vi "Enable pneumatics.vi"(8 "error in":errorcluster, 11 "UTP IO Session in":T1) -> (0 "error out":errorcluster, 3 "UTP IO Session out":T1)   [LabVIEW 2023, in "Actuators.lvlib"]
doc: "Send 1s pulse length to enable all pneumatics"
uses:
  Actuators.lvlib
  <vilib>/Noffz/UTP IO/UTP IO Library/Typedefs/Session Handle.ctl
  <vilib>/Noffz/UTP IO/UTP IO Library/UTP IO Pool Session.lvclass
  c9def3e0-2d72-4d59-8dd4-2fe76db72e2b.vi
  <vilib>/Noffz/UTP IO/UTP IO Library/methods/poly/plc/Write PLC Variable (Boolean).vi
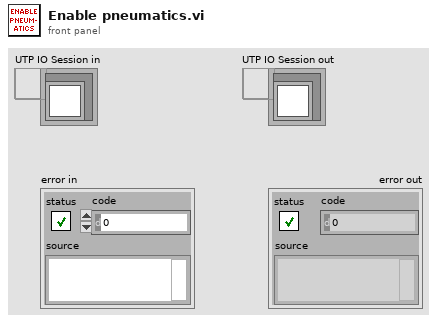
[diagram p1: front panel]
types:
  T1 = typedef "UTP IO Library.lvlib/UTP IO Pool Session.lvclass/Session Handle.ctl" = refnum<data-value>
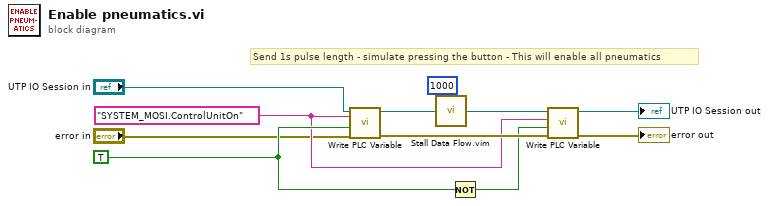
[diagram p0: block diagram]
diagram:
  w4 = TRUE ("value")
  w3 = "SYSTEM_MOSI.ControlUnitOn" ("variable name")
  # "Send 1s pulse length - simulate pressing the button - This will enable all pneumatics"
  n1 = call-poly <vilib>:"Write PLC Variable.vi"("error in (no error)"="error in", "value"=w4, "variable name"=w3, "UTP IO Session in"="UTP IO Session in") -> ("error out"=w8:errorcluster, "UTP IO Session out"=w10:T1)  [unwired: 6 in]
  n2 = call "Stall Data Flow.vim"("value in"=w10, "milliseconds to wait"=u32 1000) -> ("value out"=w9:T1)  [unwired: 1 out]
  n3 = Not(x=w4) -> (.not. x?=w6:bool)
  n4 = call-poly <vilib>:"Write PLC Variable.vi"("error in (no error)"=w8, "value"=w6, "variable name"=w3, "UTP IO Session in"=w9) -> ("error out"=→"error out":errorcluster, "UTP IO Session out"=→"UTP IO Session out":T1)  [unwired: 6 in]
